vi "EVM_5G_Sweep_Only.vi"() -> ()   [LabVIEW 2023, in "EVM.lvlib"]
uses:
  EVM.lvlib
  lib/Keysight/Keysight.lvlib
panel:
  in  "Type":enum16{"Default", "E6680A"}(ring)
  in  "Waiting Time(ms)":u32=100
  in  "FileNote":string
  out "SG Power":i32
  in  "Stop Power":i32=21
  in  "Start Power":i32=-20
  in  "SG":refnum<visa-resource-name>="TCPIP0::192.168.100.201::inst0::INSTR"
  in  "AvgTimes":i32=1
  in  "SA":refnum<visa-resource-name>="TCPIP0::192.168.100.202::inst0::INSTR"
  out "5G_EVM_Data":cluster{"X":dbl, "Y":dbl}[](graph)
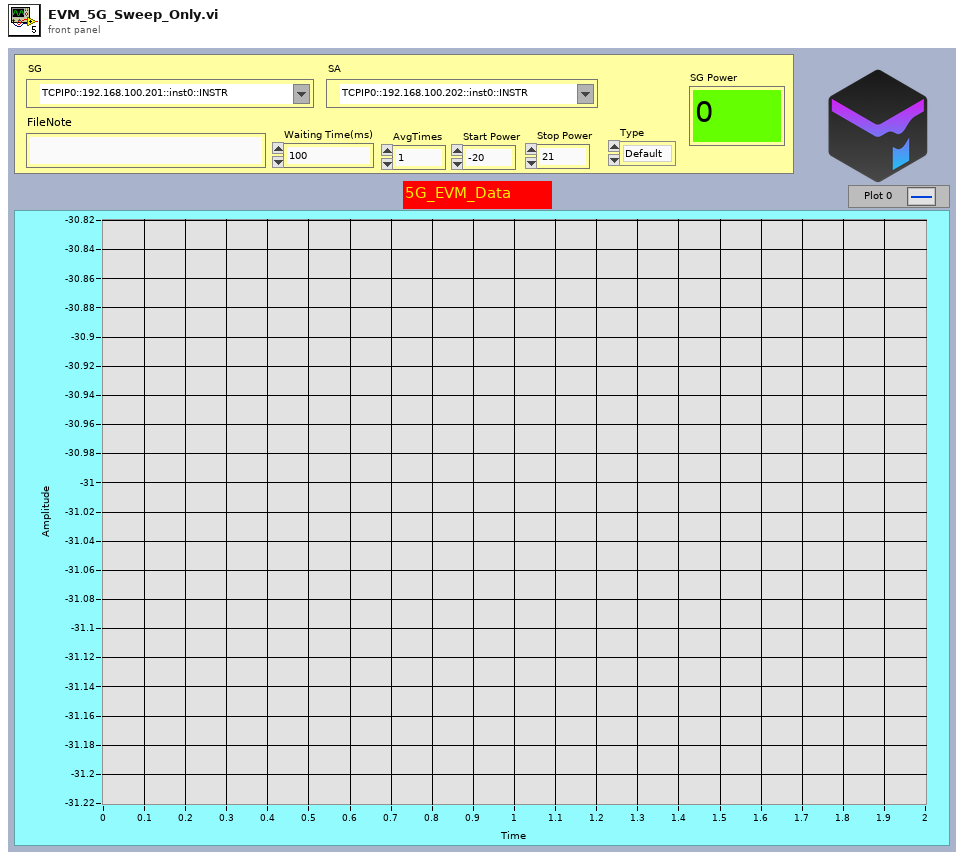
[diagram p1: front panel]
types:
  T1 = cluster{"Ch_POW_Total":dbl, "Ch_POW_Active":dbl, "EVM_RMS":dbl, "Freq_Error":dbl}
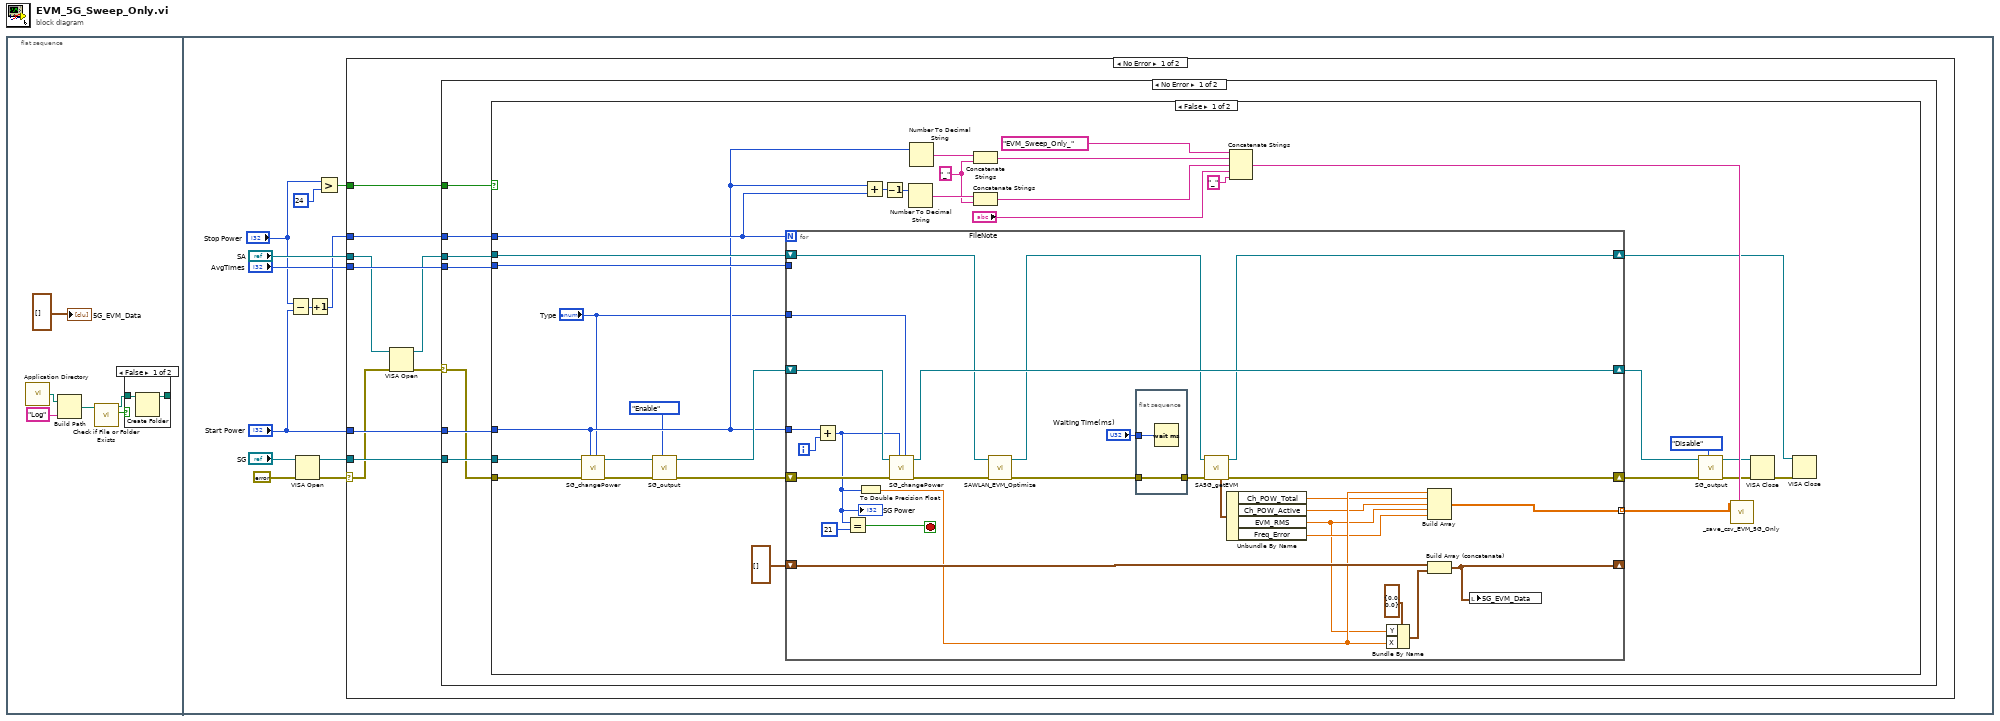
[diagram p0: block diagram]
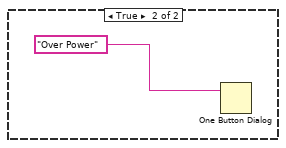
[diagram p3: hidden frame]
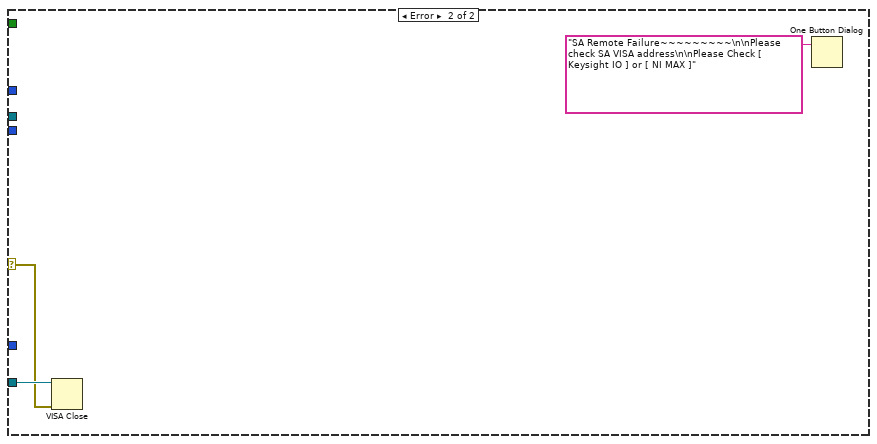
[diagram p4: hidden frame]
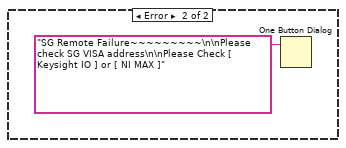
[diagram p5: hidden frame]
diagram:
  n1 = flat-sequence {
    frame #0 {
      n2 = call <vilib>:"Application Directory.vi"() -> ("Application Directory"=w5:path)
      n3 = Build Path(base path=w5, name or relative path="Log") -> (appended path=w2:path)
      n4 = call <vilib>:"Check if File or Folder Exists.vi"("path"=w2) -> ("file or folder exists?"=w4:bool, "dup path"=w3:path)  [unwired: 8 in, 1 out]
      n5 = case shown="False" w4 {
        tunnel: w3 -> [w8 w9]
        tunnel: [w7 w9] -> _
        frame False {
          n6 = Create Folder(path (use dialog)=w8) -> (created path=w7:path)  [unwired: 2 in, 2 out]
        }
        frame True {
        }
      }
      "5G_EVM_Data" <- cluster{"X":dbl, "Y":dbl}[] [] ("XY Graph")
    }
    frame #1 {
      n7 = Subtract(x="Stop Power", y="Start Power") -> (x-y=w17:i32)
      n8 = VISA Open(error in (no error)=errorcluster {"status"=FALSE, "code"=0, "source"=""}, VISA resource name="SG") -> (VISA resource name=w11:refnum<visa-resource-name>, error out=w10:errorcluster)  [unwired: 3 in]
      n9 = Increment(x=w17) -> (x+1=w16:i32)
      n10 = Greater?(x="Stop Power", y=24) -> (0:w20:bool)
      n11 = case shown="No Error" w10 {
        selector: w10 -> [w25 _]
        tunnel: "SA" -> [w23 _]
        tunnel: w20 -> [w30 _]
        tunnel: "Start Power" -> [w29 _]
        tunnel: "AvgTimes" -> [w28 _]
        tunnel: w16 -> [w27 _]
        tunnel: w11 -> [w26 _]
        frame No Error {
          n12 = VISA Open(error in (no error)=w25, VISA resource name=w23) -> (VISA resource name=w22:refnum<visa-resource-name>, error out=w24:errorcluster)  [unwired: 3 in]
          n13 = case shown="No Error" w24 {
            selector: w24 -> [w31 w101]
            tunnel: w22 -> [w37 _]
            tunnel: w30 -> [w36 _]
            tunnel: w29 -> [w35 _]
            tunnel: w28 -> [w34 _]
            tunnel: w27 -> [w33 _]
            tunnel: w26 -> [w32 w102]
            frame No Error {
              n14 = case shown="False" w36 {
                tunnel: w37 -> [w69 _]
                tunnel: w34 -> [w68 _]
                tunnel: w35 -> [w42 _]
                tunnel: w31 -> [w55 _]
                tunnel: w32 -> [w54 _]
                tunnel: w33 -> [w52 _]
                frame False {
                  w61 = "_"
                  n15 = call "SG_changePower.vi"("Type"="Type", "dBm"=w42, "error in"=w55, "VISA in"=w54) -> ("error out"=w56:errorcluster, "VISA out"=w53:refnum<visa-resource-name>)  [unwired: 5 in, 1 out]
                  n16 = call "SG_output.vi"("Func."=enum16{"Disable", "Enable"}."Enable", "error in"=w56, "VISA in"=w53) -> ("error out"=w67:errorcluster, "VISA out"=w51:refnum<visa-resource-name>)  [unwired: 7 in]
                  n17 = for {
                    N: w52 -> [_]
                    tunnel: w68 -> [_]
                    tunnel: w42 -> [w95]
                    shift-right: [w90] -> w66
                    shift-left: w67 -> [w97]
                    shift-right: [w92] -> w50
                    shift-left: w51 -> [w91]
                    shift-right: [w87] -> w43
                    shift-left: w69 -> [w79]
                    shift-right: [w83] -> _
                    shift-left: cluster{"X":dbl, "Y":dbl}[] [] ("XY Graph") -> [w85]
                    tunnel: [w77] -> w40 mode=indexing
                    tunnel: "Type" -> [w75]
                    i -> [w96]
                    stop <- w93 stop-if-true
                    n18 = Add(x=w95, y=w96) -> (x+y=w82:i32)
                    "SG Power" <- w82
                    n19 = Equal?(x=w82, y=21) -> (x = y?=w93:bool)
                    n20 = To Double Precision Float(number=w82) -> (double precision float=w76:dbl)
                    n21 = call "SG_changePower.vi"("Type"=w75, "dBm"=w82, "error in"=w97, "VISA in"=w91) -> ("error out"=w81:errorcluster, "VISA out"=w92:refnum<visa-resource-name>)  [unwired: 5 in, 1 out]
                    n22 = call "SAWLAN_EVM_Optimize.vi"("error in"=w81, "VISA in"=w79) -> ("error out"=w80:errorcluster, "VISA out"=w78:refnum<visa-resource-name>)  [unwired: 8 in]
                    n23 = flat-sequence {
                      tunnel: w80 -> [w99]
                      tunnel: [w99] -> w89
                      tunnel: "Waiting Time(ms)" -> [w98]
                      frame #0 {
                        n24 = Wait (ms)(milliseconds to wait=w98) -> ()  [unwired: 1 out]
                      }
                    }
                    n25 = call "SA5G_getEVM.vi"("error in"=w89, "VISA in"=w78) -> ("error out"=w90:errorcluster, "VISA out"=w87:refnum<visa-resource-name>, "get_EVM"=w74:T1)  [unwired: 7 in]
                    n26 = Unbundle By Name(w74) -> ("Ch_POW_Total"=w71:dbl, "Ch_POW_Active"=w73:dbl, "EVM_RMS"=w70:dbl, "Freq_Error"=w72:dbl)
                    n27 = Bundle By Name(cluster=cluster{"X":dbl, "Y":dbl} {"X"=0.0, "Y"=0.0} ("element"), "Y"=w70, "X"=w76) -> (w84:cluster{"X":dbl, "Y":dbl})
                    n28 = Build Array(w76, w71, w73, w70, w72) -> (w77:dbl[])
                    n29 = Build Array (concatenate)(w85, w84) -> (w83:cluster{"X":dbl, "Y":dbl}[])
                    n30 = local write "5G_EVM_Data"(w83) -> ()
                  }
                  n31 = Add(x=w42, y=w52) -> (x+y=w65:i32)
                  n32 = Decrement(x=w65) -> (x-1=w64:i32)
                  n33 = Number To Decimal String(number=w64) -> (decimal integer string=w62:string)  [unwired: 1 in]
                  n34 = Number To Decimal String(number=w42) -> (decimal integer string=w63:string)  [unwired: 1 in]
                  n35 = Concatenate Strings(w63, w61) -> (w59:string)
                  n36 = Concatenate Strings(w62, w61) -> (w58:string)
                  n37 = Concatenate Strings("EVM_Sweep_Only_" ("delimiter (\\t)"), w59, w58, "FileNote", "_") -> (w57:string)
                  n38 = call "SG_output.vi"("Func."=enum16{"Disable", "Enable"}."Disable", "error in"=w66, "VISA in"=w50) -> ("error out"=w46:errorcluster, "VISA out"=w45:refnum<visa-resource-name>)  [unwired: 7 in]
                  n39 = call "_save_csv_EVM_5G_Only.vi"("delimiter (\\t)"=w57, "Data"=w40) -> ()  [unwired: 9 in, 1 out]
                  n40 = VISA Close(VISA resource name=w45, error in (no error)=w46) -> (error out=w44:errorcluster)
                  n41 = VISA Close(VISA resource name=w43, error in (no error)=w44) -> ()  [unwired: 1 out]
                }
                frame True {
                  n42 = One Button Dialog(message="Over Power") -> ()  [unwired: 1 in, 1 out]
                }
              }
            }
            frame Error {
              n43 = VISA Close(VISA resource name=w102, error in (no error)=w101) -> ()  [unwired: 1 out]
              n44 = One Button Dialog(message="SA Remote Failure~~~~~~~~~\n\nPlease check SA VISA address\n\nPlease Check [ Keysight IO ] or [ NI MAX ]") -> ()  [unwired: 1 in, 1 out]
            }
          }
        }
        frame Error {
          n45 = One Button Dialog(message="SG Remote Failure~~~~~~~~~\n\nPlease check SG VISA address\n\nPlease Check [ Keysight IO ] or [ NI MAX ]") -> ()  [unwired: 1 in, 1 out]
        }
      }
    }
  }
